vi "DetectCollisionSmoother.vi"(0 "Goal":dbl[](array[numeric]), 4 "Initial State":dbl[](array[numeric]), 6 "enemy_robots":T2[](array[typedef]), 7 "Robot in":T2={"id"=0, "function"=enum."Attacker", "x"=0.0, "y"=0.0, "orientation"=0.0, "v_tangent"=0.0, "v_normal"=0.0, "v_ang"=0.0, "kick_x"=0.0, "kick_z"=0.0, "dribble"=FALSE, "Timestamp"=timestamp(0 s since 1904-01-01), "estimatives"={"est_v_tangent"=0.0, "est_v_normal"=0.0, "est_vx"=0.0, "est_vy"=0.0, "Pos Robot Est"=[]}, "dest_x_kick"=0.0, "dest_y_kick"=0.0, "Gap Coord"=[], "States"=enum."Pass", "Path "=[], "Path  Smooth"=[], "Dest"=[]}, 8 "SegmentPointB":dbl[](array[numeric]), 9 "SegmentPointA":dbl[](array[numeric]), 10 "ball":dbl[](array[numeric]), 11 "IA State":T1={"our_robots"=[], "enemy_robots"=[], "balls"=[], "geometry"={"line_width"=0, "field_length"=0, "field_width"=0, "boundary_width"=0, "referee_width"=0, "goal_width"=0, "goal_depth"=0, "goal_wall_width"=0, "center_circle_radius"=0, "defense_radius"=0, "defense_stretch"=0, "free_kick_from_defense_dist"=0, "penalty_spot_from_field_line_dist"=0, "penalty_line_from_spot_dist"=0}, "IA Judge"={"stage"="", "command"="", "our_goalie_id"=0.0, "enemy_goalie_id"=0.0, "command enum"=enum."Halt", "Time"=enum."Azul"}, "Received Timestamp"=timestamp(0 s since 1904-01-01), "Events"={"Touch"=FALSE, "Ball out"=FALSE, "id touch"=0.0, "Ball out of \nVision"=FALSE, "Ball inside \nGoalie area"=FALSE, "Robot not responding"=FALSE, "Robots responding status"=[1.0, 1.0, 1.0, 1.0, 1.0, 1.0], "Enemy Ball \nPossession"=FALSE, "Pass State"=FALSE, "id end of pass"=0.0, "Kick"=FALSE, "Id ini Possession"=0.0, "Ball Possesion"=FALSE, "Id Possesion"=0.0, "Direct Kick"=FALSE, "2nd Strk Ativo"=FALSE}}) -> (3 "Is there colision?":bool)   [LabVIEW 2018]
uses:
  Core/AI Robot.ctl
  Intel/Functions Enum.ctl
  Intel/AttackerStates.ctl
  PathDests.ctl
  PathDest.ctl
  Core/AI Input.ctl
  Core/AI Ball.ctl
  Core/Field Size.ctl
  Core/AI Judge.ctl
  Intel/Command Enum.ctl
  Util/Events/Events.ctl
panel:
  in  "our_robots":T2[](array[typedef])
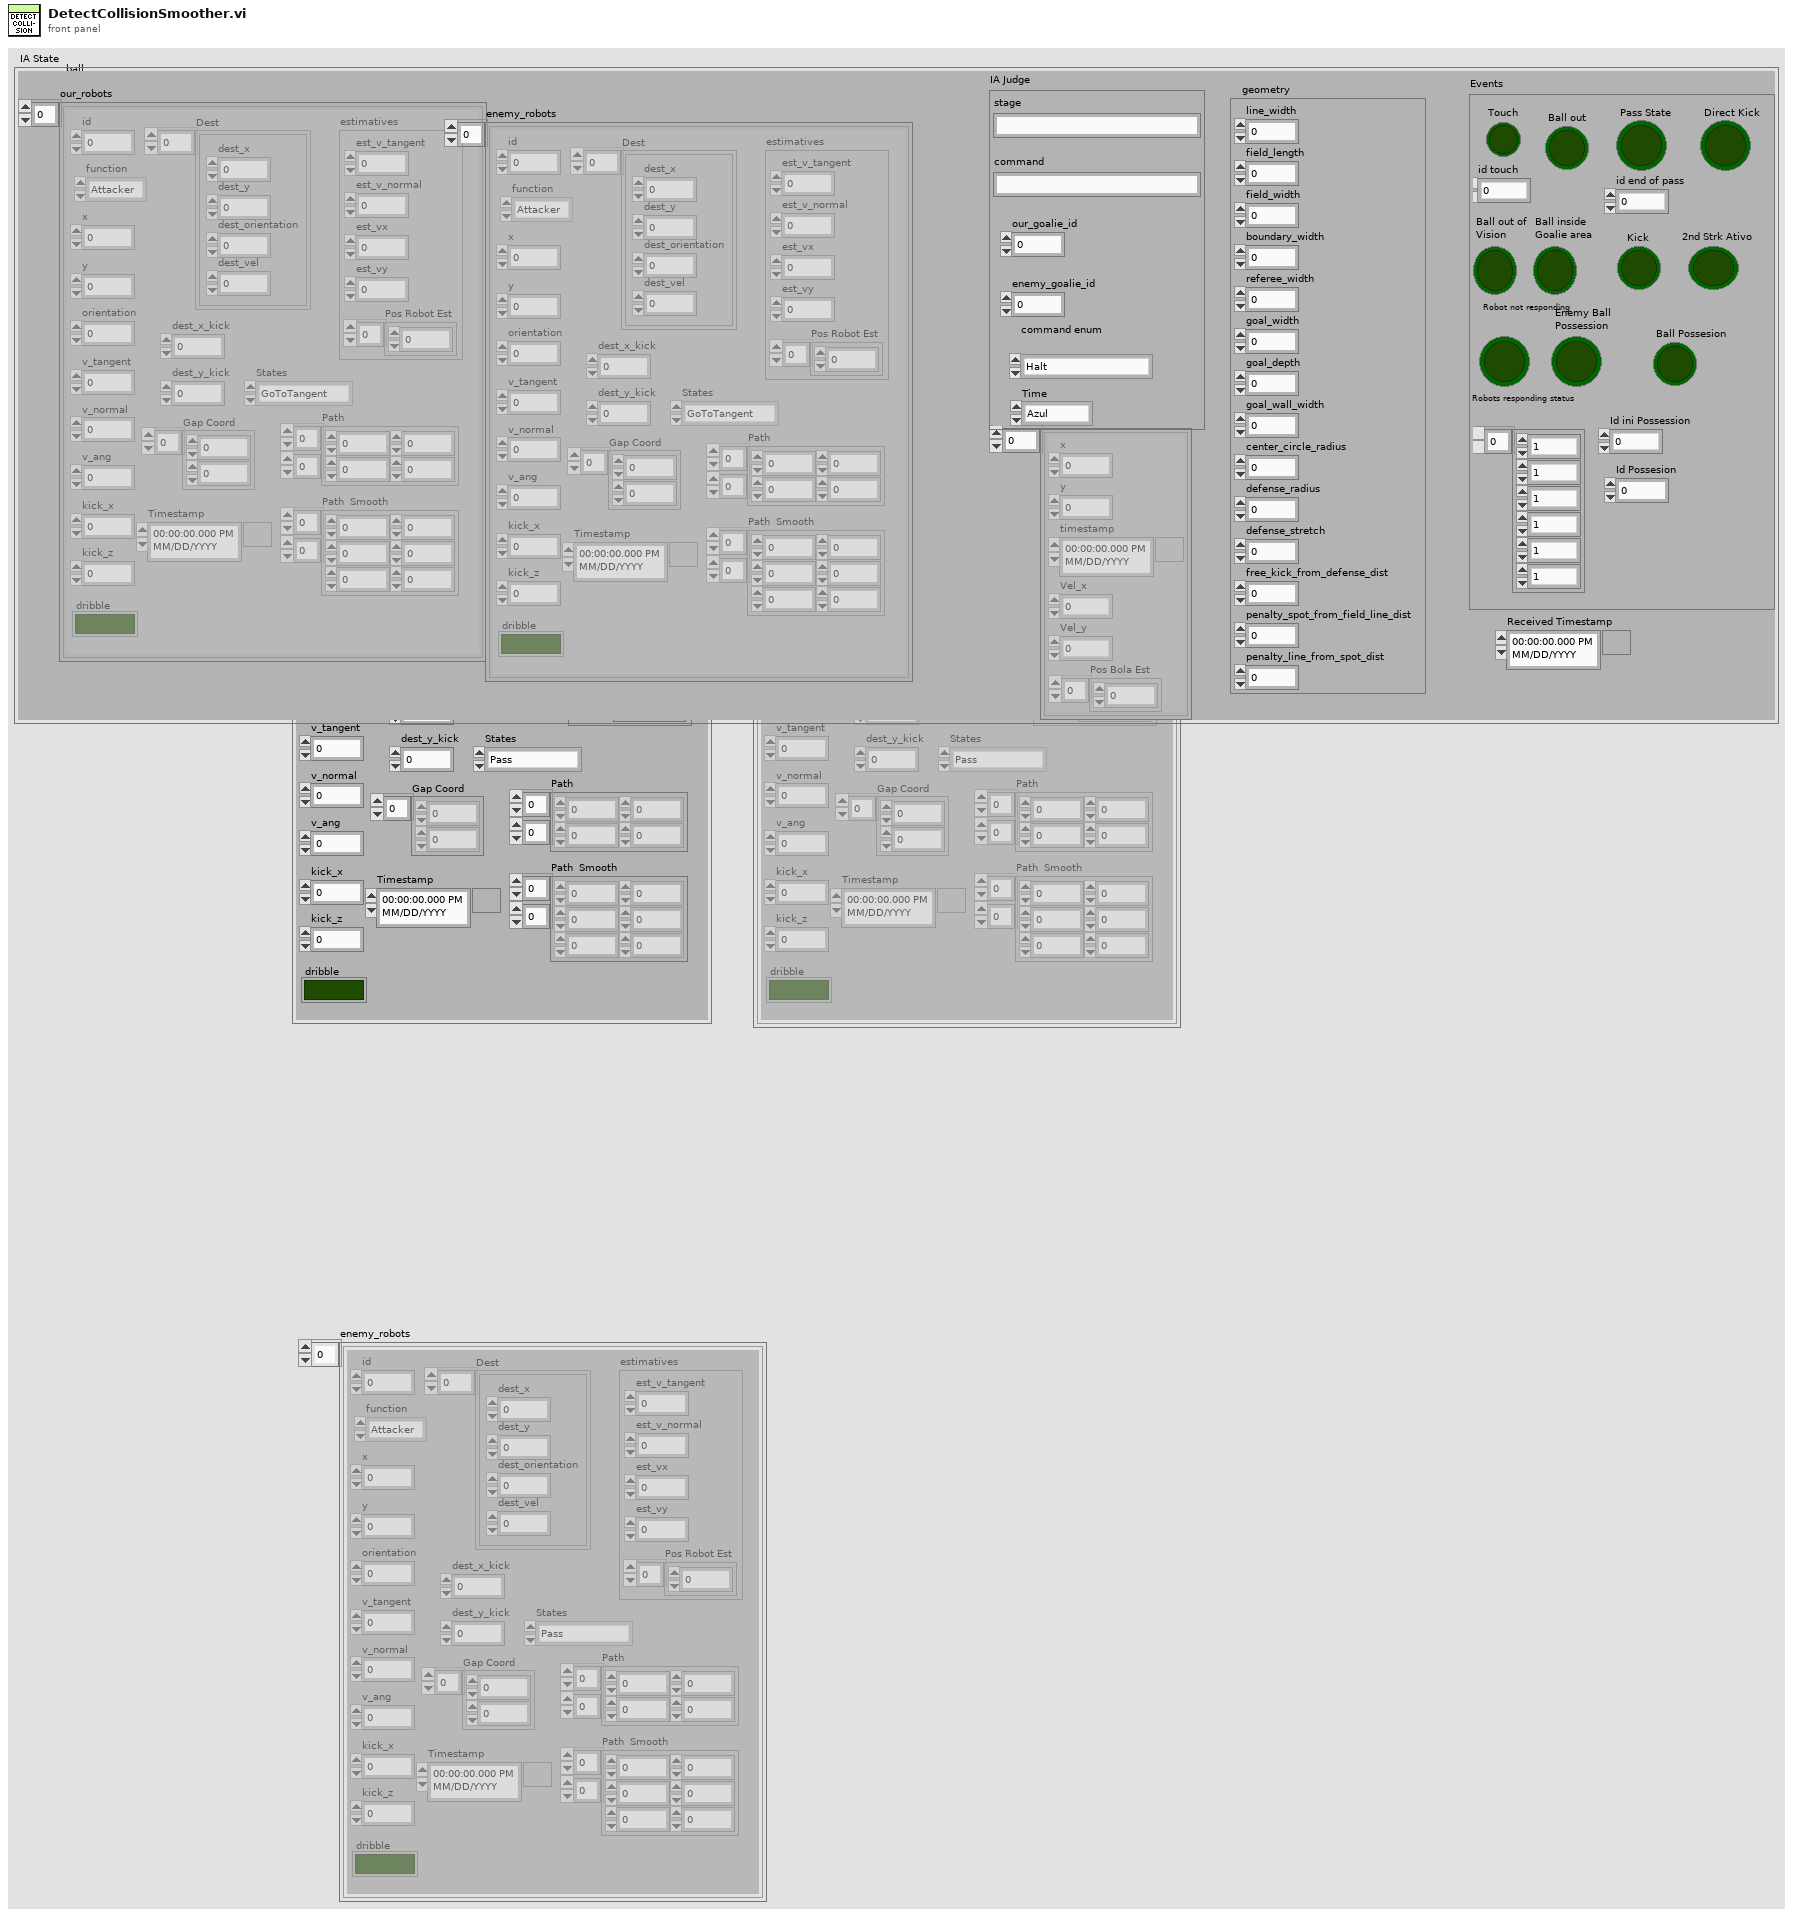
[diagram p1: front panel]
types:
  T1 = typedef "AI Input.ctl" = cluster{"our_robots":T2[], "enemy_robots":T2[], "balls":T7[], "geometry":T8, "IA Judge":T9, "Received Timestamp":timestamp, "Events":T11}
  T2 = typedef "AI Robot.ctl" = cluster{"id":u32, "function":T3, "x":dbl, "y":dbl, "orientation":dbl, "v_tangent":dbl, "v_normal":dbl, "v_ang":dbl, "kick_x":dbl, "kick_z":dbl, "dribble":bool, "Timestamp":timestamp, "estimatives":cluster{"est_v_tangent":dbl, "est_v_normal":dbl, "est_vx":dbl, "est_vy":dbl, "Pos Robot Est":dbl[]}, "dest_x_kick":dbl, "dest_y_kick":dbl, "Gap Coord":dbl[], "States":T4, "Path ":dbl[][], "Path  Smooth":dbl[][], "Dest":T5}
  T3 = typedef "Functions Enum.ctl" = enum16{"2nd Striker", "Attacker", "Goalie", "Defender", "Striker", "Goto 0", "Dummy", "Kicker", "ZigZag 0", "ZigZag 1", "ZigZag 2", "ZigZag 3", "ZigZag 4", "ZigZag 5", "ZigZag 6", "ZigZag 7", "ZigZag 8", ""}
  T4 = typedef "AttackerStates.ctl" = enum16{"Pass", "GoToTangent", "BallGetting", "GoToKick", ""}
  T5 = typedef "PathDests.ctl" = T6[]
  T6 = typedef "PathDest.ctl" = cluster{"dest_x":dbl, "dest_y":dbl, "dest_orientation":dbl, "dest_vel":dbl}
  T7 = typedef "AI Ball.ctl" = cluster{"x":dbl, "y":dbl, "timestamp":timestamp, "Vel_x":dbl, "Vel_y":dbl, "Pos Bola Est":dbl[]}
  T8 = typedef "Field Size.ctl" = cluster{"line_width":u32, "field_length":u32, "field_width":u32, "boundary_width":u32, "referee_width":u32, "goal_width":u32, "goal_depth":u32, "goal_wall_width":u32, "center_circle_radius":u32, "defense_radius":u32, "defense_stretch":u32, "free_kick_from_defense_dist":u32, "penalty_spot_from_field_line_dist":u32, "penalty_line_from_spot_dist":u32}
  T9 = typedef "AI Judge.ctl" = cluster{"stage":string, "command":string, "our_goalie_id":dbl, "enemy_goalie_id":dbl, "command enum":T10, "Time":enum16{"Azul", "Amarelo"}}
  T10 = typedef "Command Enum.ctl" = enum16{"Halt", "Stop", "Force Start", "PKA Normal Start", "Prepare Kickoff Ally", "PKE Normal Start", "Prepare Kickoff Enemy", "Prepare Penalty Ally", "PPA Normal Start", "Prepare Penalty Enemy", "PPE Normal Start", "Direct Free Enemy", "Direct Free Ally", "Indirect Free Enemy", "Indirect Free Ally", "Timeout Enemy", "Timeout Ally", "Goal Enemy", "Goal Ally", "Ball Placement Enemy", "Ball Placement Ally", "Normal Half Time", "Extra Time Break", "Extra Half Time", "None", "Post Game"}
  T11 = typedef "Events.ctl" = cluster{"Touch":bool, "Ball out":bool, "id touch":dbl, "Ball out of \nVision":bool, "Ball inside \nGoalie area":bool, "Robot not responding":bool, "Robots responding status":dbl[], "Enemy Ball \nPossession":bool, "Pass State":bool, "id end of pass":dbl, "Kick":bool, "Id ini Possession":dbl, "Ball Possesion":bool, "Id Possesion":dbl, "Direct Kick":bool, "2nd Strk Ativo":bool}
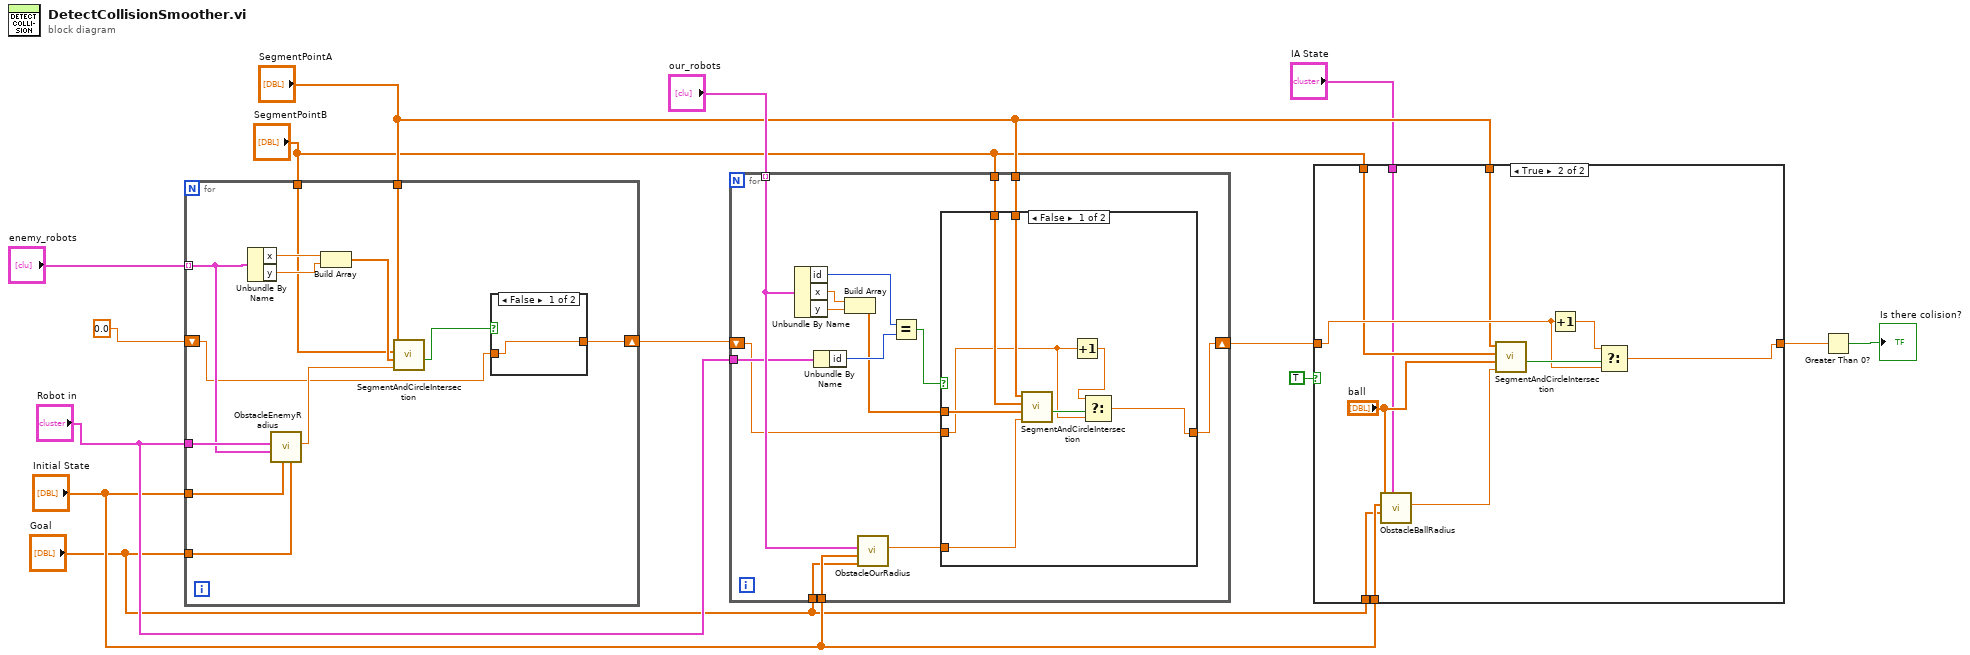
[diagram p0: block diagram]
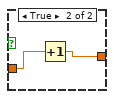
[diagram p4: hidden frame]
diagram:
  n1 = for {
    tunnel: "enemy_robots" -> [w21] mode=indexing
    tunnel: "Initial State" -> [w24]
    tunnel: "Goal" -> [w23]
    tunnel: "Robot in" -> [w22]
    tunnel: "SegmentPointA" -> [w19]
    tunnel: "SegmentPointB" -> [w18]
    shift-right: [w15] -> w10
    shift-left: 0.0 -> [w16]
    n2 = Unbundle By Name(w21) -> ("x"=w27:dbl, "y"=w26:dbl)
    n3 = call "ObstacleEnemyRadius.vi"("Goal"=w23, "Initial State"=w24, "Robot enemy"=w21, "Robot in"=w22) -> ("obstacle enemy radius"=w20:dbl)  [unwired: 7 in]
    n4 = Build Array(w27, w26) -> (w25:dbl[])
    n5 = call "SegmentAndCircleIntersection.vi"("CircleRadius"=w20, "CircleCenter"=w25, "SegmentPointB"=w18, "SegmentPointA"=w19) -> ("DoTheyIntersect?"=w17:bool)  [unwired: 7 in]
    n6 = case shown="False" w17 {
      tunnel: w16 -> [w28 w30]
      tunnel: [w28 w29] -> w15
      frame False {
      }
      frame True {
        n7 = Increment(x=w30) -> (x+1=w29:dbl)
      }
    }
  }
  n8 = for {
    tunnel: "our_robots" -> [w45] mode=indexing
    shift-right: [w38] -> w6
    shift-left: w10 -> [w37]
    tunnel: "Initial State" -> [w44]
    tunnel: "Goal" -> [w43]
    tunnel: "Robot in" -> [w42]
    tunnel: "SegmentPointA" -> [w35]
    tunnel: "SegmentPointB" -> [w34]
    n9 = Unbundle By Name(w45) -> ("id"=w41:u32, "x"=w33:dbl, "y"=w32:dbl)
    n10 = Unbundle By Name(w42) -> ("id"=w40:u32)
    n11 = Build Array(w33, w32) -> (w31:dbl[])
    n12 = call "ObstacleOurRadius.vi"("Goal"=w43, "Initial State"=w44, "other robot"=w45) -> ("obstacle enemy radius"=w36:dbl)  [unwired: 8 in]
    n13 = Equal?(x=w41, y=w40) -> (x = y?=w39:bool)
    n14 = case shown="False" w39 {
      tunnel: [w47 w54] -> w38
      tunnel: w37 -> [w46 w54]
      tunnel: w36 -> [w53 _]
      tunnel: w35 -> [w52 _]
      tunnel: w34 -> [w51 _]
      tunnel: w31 -> [w50 _]
      frame False {
        n15 = call "SegmentAndCircleIntersection.vi"("CircleRadius"=w53, "CircleCenter"=w50, "SegmentPointB"=w51, "SegmentPointA"=w52) -> ("DoTheyIntersect?"=w49:bool)  [unwired: 7 in]
        n16 = Increment(x=w46) -> (x+1=w48:dbl)
        n17 = Select(t=w48, s=w49, f=w46) -> (s? t:f=w47:dbl)
      }
      frame True {
      }
    }
  }
  n18 = case shown="True" TRUE {
    tunnel: [w55 w60] -> w7
    tunnel: w6 -> [w55 w61]
    tunnel: "Initial State" -> [_ w66]
    tunnel: "Goal" -> [_ w65]
    tunnel: "SegmentPointA" -> [_ w59]
    tunnel: "SegmentPointB" -> [_ w58]
    tunnel: "IA State" -> [_ w56]
    frame False {
    }
    frame True {
      n19 = call "ObstacleBallRadius.vi"("IA State"=w56, "Goal"=w65, "Initial State"=w66, "ball"="ball") -> ("obstacle ball radius"=w64:dbl)  [unwired: 7 in]
      n20 = call "SegmentAndCircleIntersection.vi"("CircleRadius"=w64, "CircleCenter"="ball", "SegmentPointB"=w58, "SegmentPointA"=w59) -> ("DoTheyIntersect?"=w63:bool)  [unwired: 7 in]
      n21 = Increment(x=w61) -> (x+1=w62:dbl)
      n22 = Select(t=w62, s=w63, f=w61) -> (s? t:f=w60:dbl)
    }
  }
  n23 = Greater Than 0?(x=w7) -> (x > 0?=→"Is there colision?":bool)
